vi "Generate Waveform.vi"(8 "error in (no error)":errorcluster, 11 "Waveform in":refnum<class "Waveform.lvclass">) -> (0 "error out":errorcluster, 3 "Waveform out":refnum<class "Waveform.lvclass">)   [LabVIEW 2011, in "Waveform.lvclass"]
uses:
  Waveform.lvclass
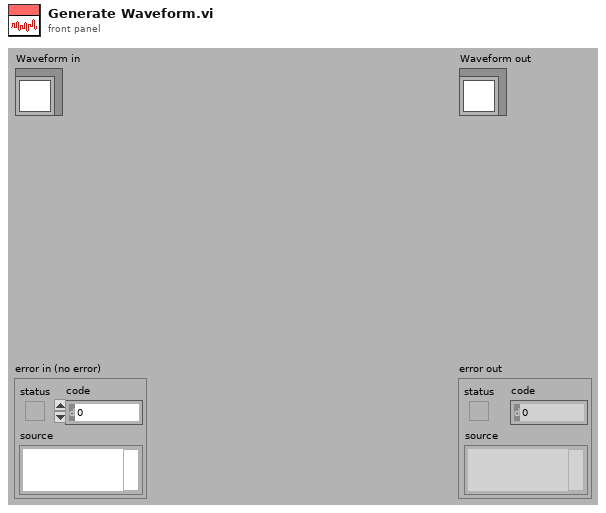
[diagram p1: front panel]
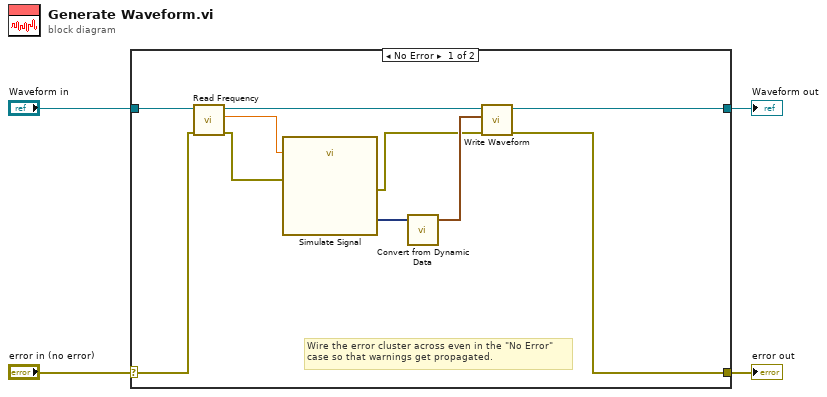
[diagram p0: block diagram]
diagram:
  n1 = case shown="No Error" "error in (no error)" {
    selector: "error in (no error)" -> [w6 w16]
    tunnel: [w5 w16] -> w3
    tunnel: [w7 w15] -> w1
    tunnel: "Waveform in" -> [w8 w15]
    frame No Error {
      # "Wire the error cluster across even in the \"No Error\"\ncase so that warnings get propagated."
      n2 = call-dynamic "Read Frequency.vi"("error in (no error)"=w6, "Waveform in"=w8) -> ("error out"=w12:errorcluster, "Frequency"=w14:dbl, "Waveform out"=w11:refnum<class "Waveform.lvclass">)  [unwired: 7 in]
      n3 = call "Simulate Signal"("Frequency"=w14, "error in (no error)"=w12) -> ("Sine"=w13:dynamicdata, "error out"=w9:errorcluster)  [unwired: 12 in]
      n4 = call "Convert from Dynamic Data"("Dynamic Data Type"=w13) -> ("Waveform"=w10:waveform(dbl))  [unwired: 3 in]
      n5 = call-dynamic "Write Waveform.vi"("error in (no error)"=w9, "Waveform"=w10, "Waveform in"=w11) -> ("error out"=w5:errorcluster, "Waveform out"=w7:refnum<class "Waveform.lvclass">)  [unwired: 7 in]
    }
    frame Error {
    }
  }
  "error out" <- w3
  "Waveform out" <- w1
